vi "initialise.vi"(8 "error in (no error)":errorcluster, 11 "GenericPlugin in":refnum<class "StimulatorDL090503.lvclass">) -> (0 "error out":errorcluster, 3 "GenericPlugin out":refnum<class "StimulatorDL090503.lvclass">)   [LabVIEW 2010, in "StimulatorDL090503.lvclass"]
doc: "The dynamic dispatch-version of this VI initalises the plug-in object by allocating and initalising any dynamic resources need."
uses:
  StimulatorDL090503.lvclass
  StimulatorDL090503Scaffold/StimulatorDL090503Scaffold/StimulatorDL090503Scaffold.lvclass
  common/enumerations/functional_global_action_enum.ctl
  StimulatorDL090503.lvclass/StimulatorDL090503.ctl
  SignalWriter/GenericSignalWriter/GenericSignalWriter/GenericSignalWriter.lvclass
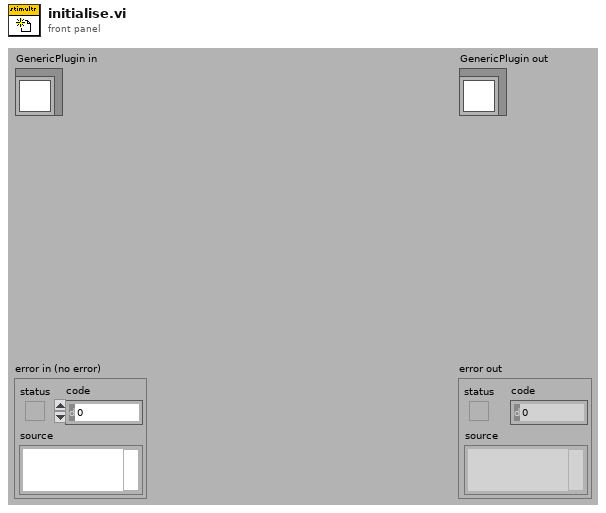
[diagram p1: front panel]
types:
  T1 = typedef "functional_global_action_enum.ctl" = enum16{"get", "set", "reset"}
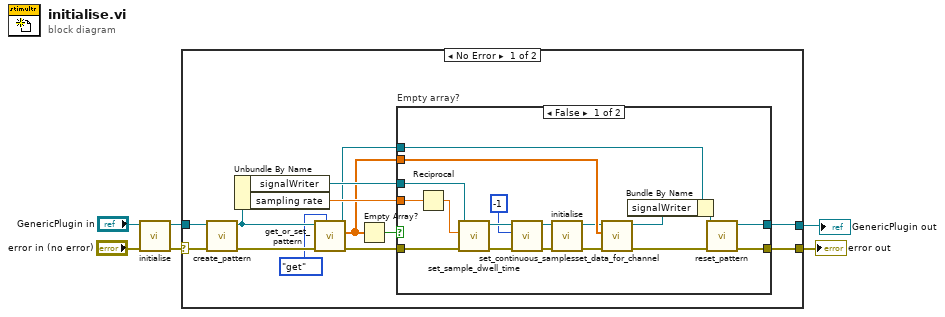
[diagram p0: block diagram]
diagram:
  n1 = call-parent "initialise.vi"("error in (no error)"="error in (no error)", "GenericPlugin in"="GenericPlugin in") -> ("error out"=w4:errorcluster, "GenericPlugin out"=w3:refnum<class "StimulatorDL090503.lvclass">)  [unwired: 8 in]
  n2 = case shown="No Error" w4 {
    selector: w4 -> [w16 w40]
    tunnel: w3 -> [w15 w41]
    tunnel: [w19 w40] -> w2
    tunnel: [w17 w41] -> w1
    frame No Error {
      n3 = call "create_pattern.vi"("error in (no error)"=w16, "StimulatorDL090503 in"=w15) -> ("error out"=w11:errorcluster, "StimulatorDL090503 out"=w9:refnum<class "StimulatorDL090503.lvclass">)  [unwired: 8 in]
      n4 = Unbundle By Name(w9) -> ("signalWriter"=w14:refnum<class "GenericSignalWriter.lvclass">, "sampling rate"=w13:dbl[unit])
      n5 = call "get_or_set_pattern.vi"("action"=functional_global_action_enum."get", "error in (no error)"=w11, "StimulatorDL090503 in"=w9) -> ("error out"=w10:errorcluster, "pattern out"=w12:dbl[], "StimulatorDL090503 out"=w8:refnum<class "StimulatorDL090503.lvclass">)  [unwired: 6 in]
      n6 = Empty Array?(array=w12) -> (empty?=w18:bool)
      n7 = case "Empty array?" shown="False" w18 {
        tunnel: w10 -> [w27 w39]
        tunnel: [w24 w39] -> w19
        tunnel: w8 -> [w22 w38]
        tunnel: [w23 w38] -> w17
        tunnel: w12 -> [w30 _]
        tunnel: w14 -> [w26 _]
        tunnel: w13 -> [w32 _]
        frame False {
          n8 = Reciprocal(x=w32) -> (1/x=w31:dbl[unit])
          n9 = call-dynamic "set_sample_dwell_time.vi"("error in (no error)"=w27, "sample dwell time"=w31, "GenericWriteSignals.lvclass in"=w26) -> ("error out"=w37:errorcluster, "GenericWriteSignals.lvclass out"=w36:refnum<class "GenericSignalWriter.lvclass">)  [unwired: 7 out]
          n10 = call-dynamic "set_continuous_samples.vi"("error in (no error)"=w37, "continuous samples"=-1, "GenericWriteSignals.lvclass in"=w36) -> ("error out"=w34:errorcluster, "GenericWriteSignals.lvclass out"=w35:refnum<class "GenericSignalWriter.lvclass">)  [unwired: 7 out]
          n11 = call-dynamic "initialise.vi"("error in (no error)"=w34, "GenericPlugin in"=w35) -> ("error out"=w28:errorcluster, "GenericPlugin out"=w29:refnum<class "GenericSignalWriter.lvclass">)  [unwired: 8 out]
          n12 = call-dynamic "set_data_for_channel.vi"("error in (no error)"=w28, "data"=w30, "GenericWriteSignals in"=w29) -> ("error out"=w25:errorcluster, "GenericWriteSignals out"=w21:refnum<class "GenericSignalWriter.lvclass">)  [unwired: 7 out]
          n13 = Bundle By Name(cluster=w22, "signalWriter"=w21) -> (w20:refnum<class "StimulatorDL090503.lvclass">)
          n14 = call "reset_pattern.vi"("error in (no error)"=w25, "StimulatorDL090503 in"=w20) -> ("error out"=w24:errorcluster, "StimulatorDL090503 out"=w23:refnum<class "StimulatorDL090503.lvclass">)  [unwired: 8 in]
        }
        frame True {
        }
      }
    }
    frame Error {
    }
  }
  "error out" <- w2
  "GenericPlugin out" <- w1
